vi "TS Start DAC Init.vi"(8 "error in":errorcluster, 11 "Test Stand in":refnum<class "Generic Test Stand.lvclass">) -> (0 "error out":errorcluster, 3 "Test Stand out":refnum<class "Generic Test Stand.lvclass">)   [LabVIEW 2019, in "Generic Test Stand.lvclass"]
uses:
  Generic Test Stand.lvclass
  Generic Test Stand.lvclass/Generic Test Stand.ctl
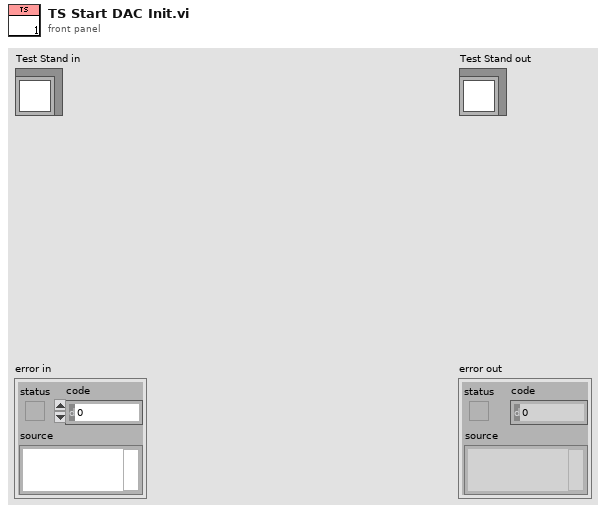
[diagram p1: front panel]
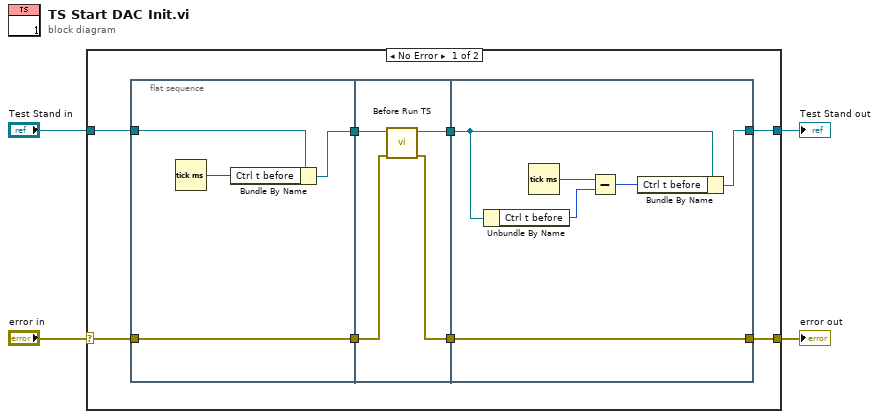
[diagram p0: block diagram]
diagram:
  n1 = case shown="No Error" "error in" {
    selector: "error in" -> [w8 w28]
    tunnel: [w5 w28] -> w3
    tunnel: [w9 w27] -> w1
    tunnel: "Test Stand in" -> [w12 w27]
    frame No Error {
      n2 = flat-sequence {
        tunnel: w12 -> [w15]
        tunnel: [w14] -> w11
        tunnel: w8 -> [w13]
        tunnel: [w13] -> w7
        tunnel: w11 -> [w20]
        tunnel: [w19] -> w10
        tunnel: w7 -> [w18]
        tunnel: [w17] -> w6
        tunnel: w10 -> [w22]
        tunnel: [w24] -> w9
        tunnel: w6 -> [w21]
        tunnel: [w21] -> w5
        frame #0 {
          n3 = Tick Count (ms)() -> (millisecond timer value=w16:u32)
          n4 = Bundle By Name(cluster=w15, "Ctrl t before"=w16) -> (w14:refnum<class "Generic Test Stand.lvclass">)
        }
        frame #1 {
          n5 = call-dynamic "Before Run TS.vi"("error in"=w18, "Test Stand in"=w20) -> ("error out"=w17:errorcluster, "Test Stand out"=w19:refnum<class "Generic Test Stand.lvclass">)  [unwired: 8 in]
        }
        frame #2 {
          n6 = Unbundle By Name(w22) -> ("Ctrl t before"=w26:u32)
          n7 = Tick Count (ms)() -> (millisecond timer value=w25:u32)
          n8 = Subtract(x=w25, y=w26) -> (x-y=w23:u32)
          n9 = Bundle By Name(cluster=w22, "Ctrl t before"=w23) -> (w24:refnum<class "Generic Test Stand.lvclass">)
        }
      }
    }
    frame Error {
    }
  }
  "error out" <- w3
  "Test Stand out" <- w1
